vi "InitWebsocketMessageBroker.vi"(8 "error in (no error)":errorcluster, 9 "Listen Port":u16, 10 "Websocket Topic Actor":refnum<class "Websocket Topic Actor.lvclass">, 11 "Broker Name":string) -> (0 "error out":errorcluster, 3 "Message Broker Ref":refnum<data-value>)   [LabVIEW 2016, in "Stream Mediator.lvlib" / "Websocket Message Broker.lvclass"]
doc: "--\nCopyright © 2017 Composed SystemsI All rights reserved.\n\nAuthor: Jon McBee <jon.mcbee@composed.io>\n\nThis library is provided \"AS IS\" ,WITHOUT WARRANTIES OR\nCONDITIONS OF ANY KIND, either express or implied.\n\nComposed Systems -- composed.io\n\nStream 0.0.1.1\nJon McBee - Composed Systems\nCopyright (c) 2017, Composed Systems"
uses:
  <userlib>/Composed Systems/Stream/Mediator/Classes/Websocket Message Broker/Websocket Message Broker.lvclass
  <userlib>/Composed Systems/Stream/Mediator/Classes/Websocket Topic Actor/Websocket Topic Actor.lvclass
  C:/Program Files (x86)/National Instruments/LabVIEW 2016/user.lib/Composed Systems/Stream/Mediator/Classes/Topic Actor/Topic Actor.lvclass
  C:/Program Files (x86)/National Instruments/LabVIEW 2016/user.lib/Composed Systems/Stream/Mediator/Classes/Message Broker/Message Broker.lvclass
  <userlib>/Composed Systems/Stream/Mediator/Classes/Topic Actor Look Up Table/Topic Actor Look Up Table.lvclass
  <userlib>/Composed Systems/Stream/Mediator/Classes/Websocket Message Broker/Websocket Message Broker.lvclass/Websocket Message Broker.ctl
  <userlib>/Composed Systems/Stream/Mediator/Classes/Message Broker/Message Broker.lvclass
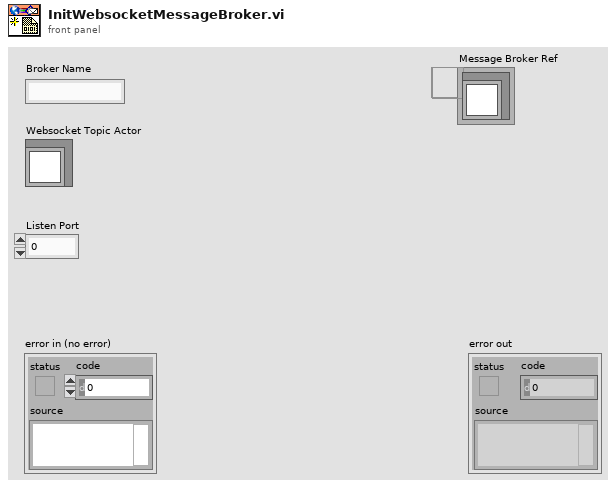
[diagram p1: front panel]
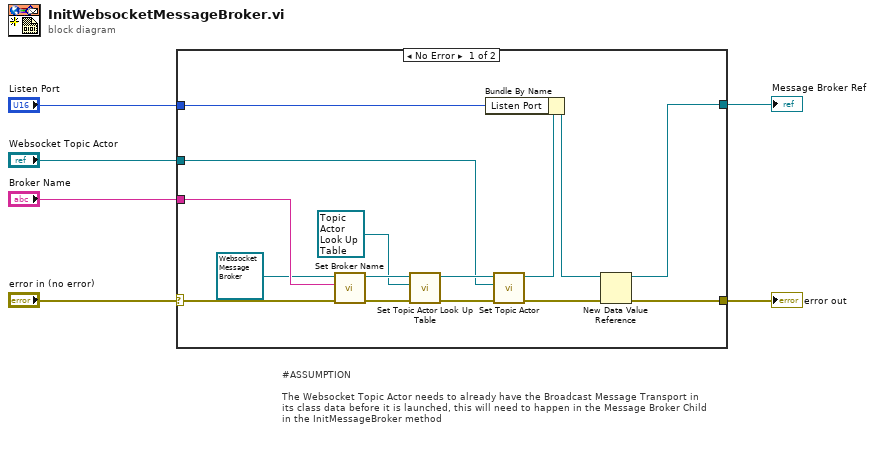
[diagram p0: block diagram]
diagram:
  # "#ASSUMPTION\n\nThe Websocket Topic Actor needs to already have the Broadcast Message Transport in\nits class data before it is launched, this will need to happen in the Message Broker Child\nin the InitMessageBroker method"
  n1 = case shown="No Error" "error in (no error)" {
    selector: "error in (no error)" -> [w13 w22]
    tunnel: [w16 w22] -> w5
    tunnel: "Websocket Topic Actor" -> [w7 _]
    tunnel: "Broker Name" -> [w21 _]
    tunnel: "Listen Port" -> [w20 _]
    tunnel: [w15 _] -> w1
    frame No Error {
      n2 = call <userlib>:"Set Broker Name.vi"("error in (no error)"=w13, "Broker Name"=w21, "Message Broker in"=refnum<class "Websocket Message Broker.lvclass"> refnum ("Websocket Message Broker in")) -> ("error out"=w18:errorcluster, "Message Broker out"=w19:refnum<class "Websocket Message Broker.lvclass">)  [unwired: 7 in]
      n3 = call <userlib>:"Set Topic Actor Look Up Table.vi"("error in (no error)"=w18, "Topic Actor Look Up Table"=refnum<class "Topic Actor Look Up Table.lvclass"> refnum, "Message Broker in"=w19) -> ("error out"=w8:errorcluster, "Message Broker out"=w9:refnum<class "Websocket Message Broker.lvclass">)  [unwired: 7 in]
      n4 = call-dynamic "Set Topic Actor.vi"("error in (no error)"=w8, "Topic Actor"=w7, "Message Broker in"=w9) -> ("error out"=w11:errorcluster, "Message Broker out"=w10:refnum<class "Websocket Message Broker.lvclass">)  [unwired: 7 in]
      n5 = Bundle By Name(cluster=w10, "Listen Port"=w20) -> (w14:refnum<class "Websocket Message Broker.lvclass">)
      n6 = New Data Value Reference(data value=w14, error in=w11) -> (data value reference=w15:refnum<data-value>, error out=w16:errorcluster)
    }
    frame Error {
    }
  }
  "error out" <- w5
  "Message Broker Ref" <- w1
